vi "LS372_read_only_Split_Cluster.vi"(0 "LS372_only_read-Cluster":T1) -> (1 "LS372_only_read-Cluster Status":T3, 2 "LS372_only_read-Cluster Control":T2)   [LabVIEW 2019]
uses:
  LS372/LS372_read_only-Status.ctl
  LS372/LS372_read_only-Control.ctl
  LS372/LS372_read_only-Cluster.ctl
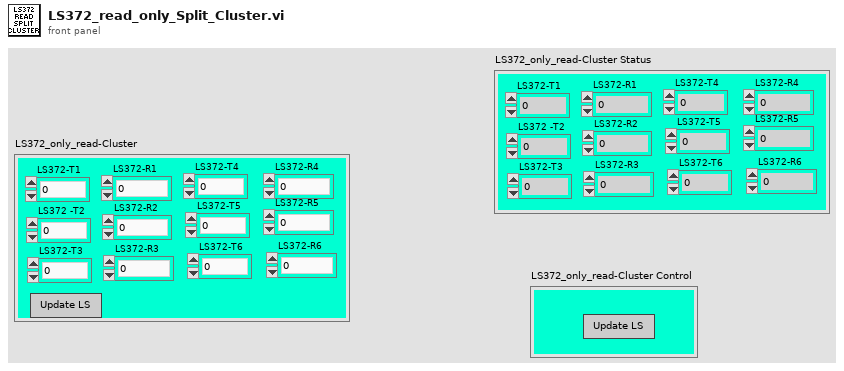
[diagram p1: front panel]
types:
  T1 = typedef "LS372_read_only-Cluster.ctl" = cluster{"LS372-T1":dbl, "LS372 -T2":dbl, "LS372-T4":dbl, "LS372-T5":dbl, "LS372-T6":dbl, "LS372-R1 ":dbl, "LS372-R2":dbl, "LS372-R3 ":dbl, "LS372-R4 \n\n\n\n":dbl, "LS372-R5":dbl, "LS372-R6 ":dbl, "LS372-T3":dbl, "Update Lakeshores":bool}
  T2 = typedef "LS372_read_only-Control.ctl" = cluster{"Update Lakeshores":bool}
  T3 = typedef "LS372_read_only-Status.ctl" = cluster{"LS372-T1":dbl, "LS372 -T2":dbl, "LS372-T4":dbl, "LS372-T5":dbl, "LS372-T6":dbl, "LS372-R1 ":dbl, "LS372-R2":dbl, "LS372-R3 ":dbl, "LS372-R4 \n\n\n\n":dbl, "LS372-R5":dbl, "LS372-R6 ":dbl, "LS372-T3":dbl}
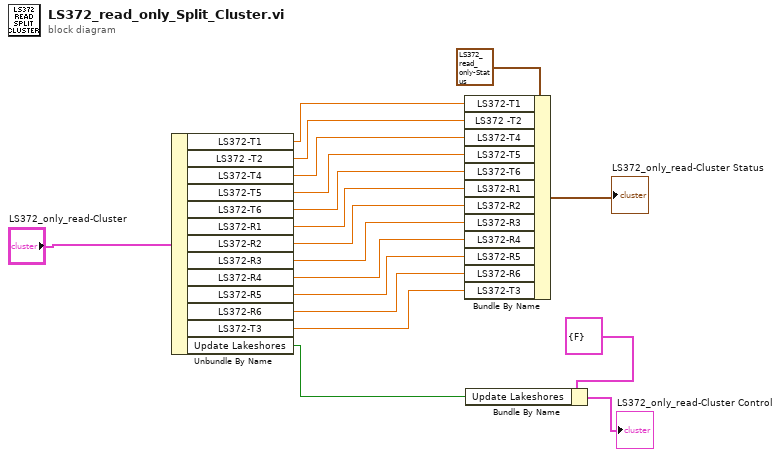
[diagram p0: block diagram]
diagram:
  n1 = Unbundle By Name("LS372_only_read-Cluster") -> ("LS372-T1"=w14:dbl, "LS372 -T2"=w13:dbl, "LS372-T4"=w12:dbl, "LS372-T5"=w11:dbl, "LS372-T6"=w10:dbl, "LS372-R1"=w9:dbl, "LS372-R2"=w8:dbl, "LS372-R3"=w7:dbl, "LS372-R4"=w6:dbl, "LS372-R5"=w5:dbl, "LS372-R6"=w4:dbl, "LS372-T3"=w3:dbl, "Update Lakeshores"=w2:bool)
  n2 = Bundle By Name(cluster=T3 {"LS372-T1"=0.0, "LS372 -T2"=0.0, "LS372-T4"=0.0, "LS372-T5"=0.0, "LS372-T6"=0.0, "LS372-R1 "=0.0, "LS372-R2"=0.0, "LS372-R3 "=0.0, "LS372-R4 \n\n\n\n"=0.0, "LS372-R5"=0.0, "LS372-R6 "=0.0, "LS372-T3"=0.0} ("LS372_only_read-Cluster Status 2"), "LS372-T1"=w14, "LS372 -T2"=w13, "LS372-T4"=w12, "LS372-T5"=w11, "LS372-T6"=w10, "LS372-R1"=w9, "LS372-R2"=w8, "LS372-R3"=w7, "LS372-R4"=w6, "LS372-R5"=w5, "LS372-R6"=w4, "LS372-T3"=w3) -> (→"LS372_only_read-Cluster Status":T3)
  n3 = Bundle By Name(cluster=T2 {"Update Lakeshores"=FALSE} ("LS372_only_read-Cluster Control"), "Update Lakeshores"=w2) -> (→"LS372_only_read-Cluster Control":T2)
